vi "stage_move_absolute.vi"(7 "Stage Name":string, 8 "error in (no error)":errorcluster, 9 "wait_for_done":bool, 10 "Position":dbl, 11 "mcl_piezo in":refnum<class "mcl_piezo.lvclass">) -> (0 "error out":errorcluster, 3 "mcl_piezo out":refnum<class "mcl_piezo.lvclass">)   [LabVIEW 2015, in "mcl_piezo.lvclass"]
uses:
  mcl_piezo.lvclass
  mcl_piezo.lvclass/mcl_piezo.ctl
  Madlib.dll
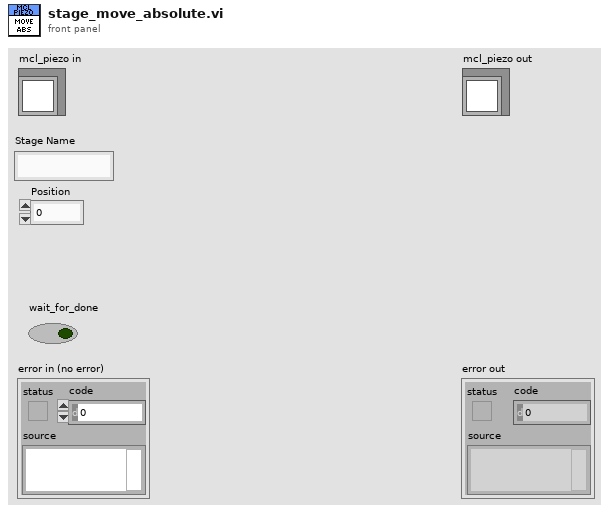
[diagram p1: front panel]
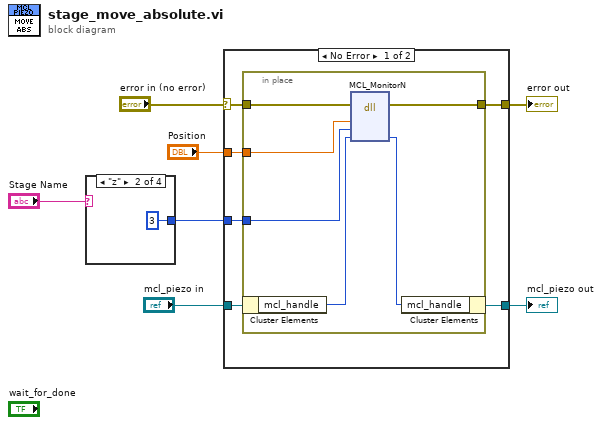
[diagram p0: block diagram]
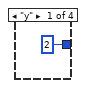
[diagram p2: hidden frame]
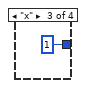
[diagram p3: hidden frame]
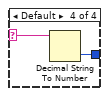
[diagram p4: hidden frame]
diagram:
  n1 = case shown="\"z\"" "Stage Name" {
    selector: "Stage Name" -> [_ _ _ w12]
    tunnel: [2 3 1 w11] -> w1
    frame "y" {
    }
    frame "z" {
    }
    frame "x" {
    }
    frame Default {
      n2 = Decimal String To Number(string=w12) -> (number=w11:i32)  [unwired: 2 in, 1 out]
    }
  }
  n3 = case shown="No Error" "error in (no error)" {
    selector: "error in (no error)" -> [w15 w26]
    tunnel: "mcl_piezo in" -> [w18 w25]
    tunnel: [w17 w25] -> w5
    tunnel: w1 -> [w16 _]
    tunnel: "Position" -> [w14 _]
    tunnel: [w13 w26] -> w3
    frame No Error {
      n4 = in-place {
        in-place-border: w16 -> [w23]
        in-place-border: w15 -> [w24]
        in-place-border: w14 -> [w22]
        in-place-border: [w19] -> w13
        n5 = in-place-cluster #1(w18) -> ("mcl_handle"=w21:i32)
        n6 = dll-call lib="C:/Users/bspoka/Documents/LabVIEW Data/lview_180307/Stage Class/MCL_3d200/MADLib.dll" fn="MCL_MonitorN"(error in=w24, "position"=w22, "axis"=w23, "handle"=w21) -> (error out=w19:errorcluster, "handle"=w20:i32)  [unwired: 5 in, 1 out]
        n7 = in-place-cluster #1("mcl_handle"=w20) -> (w17:refnum<class "mcl_piezo.lvclass">)
      }
    }
    frame Error {
    }
  }
  "error out" <- w3
  "mcl_piezo out" <- w5
